vi "Get Lines.vi"(6 "Start of Commands":string, 9 "Auto File":path=path "C:/Users/theST/Desktop/Test.txt") -> (1 "Lines":string[](array[string]), 3 "Lines of File":i32)   [LabVIEW 2016]
uses:
  <vilib>/Utility/file.llb/Read Delimited Spreadsheet (string).vi
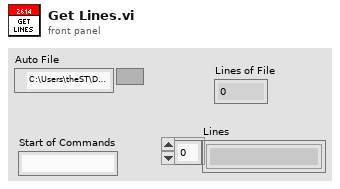
[diagram p1: front panel]
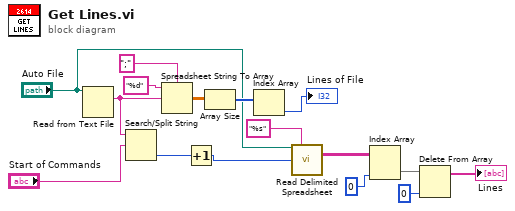
[diagram p0: block diagram]
diagram:
  n1 = Read from Text File(file (use dialog)="Auto File") -> (text=w9:string)  [unwired: 3 in, 3 out]
  n2 = Search/Split String(string=w9, search string/char (-)="Start of Commands") -> (offset of match=w6:i32)  [unwired: 1 in, 2 out]
  n3 = Spreadsheet String To Array(delimiter (Tab)=";" ("format string"), format string="%d", spreadsheet string=w9) -> (array=w15:dbl[][])  [unwired: 1 in]
  n4 = Increment(x=w6) -> (x+1=w4:i32)
  n5 = Array Size(array=w15) -> (size(s)=w10:i32[])
  n6 = Index Array(array=w10) -> (element=→"Lines of File":i32)  [unwired: 1 in]
  n7 = call-poly <vilib>:"Read Delimited Spreadsheet.vi"("file path (dialog if empty)"="Auto File", "format (%s)"="%s", "start of read offset (chars.:0)"=w4) -> ("all rows"=w12:string[][])  [unwired: 7 in, 5 out]
  n8 = Index Array(array=w12, index (col)=0 ("disabled index (col)")) -> (element=w3:string[])  [unwired: 1 in]
  n9 = Delete From Array(array=w3, index=0) -> (array with subset deleted=→"Lines":string[])  [unwired: 1 in, 1 out]
